vi "Periodic Tasks.vi"(8 "error in":errorcluster) -> ()   [LabVIEW 2020]
doc: "This VI runs in parallel to other robot code. It can contain as many user-defined periodic loops as you need. These can carry out PID or other sorts of timed response."
uses:
  <vilib>/Rock Robotics/WPI/ThirdParty/Phoenix-LabVIEW/Motor Controller/Get/CTRE_Phoenix_MotorController_GetSupplyAndStatorCurrent_Enhanced.vi
  <vilib>/Rock Robotics/WPI/ThirdParty/Phoenix-LabVIEW/Motor Controller/Get/CTRE_Phoenix_MotorController_GetSelectedSensorData.vi
  <vilib>/Rock Robotics/WPI/ThirdParty/Phoenix-LabVIEW/Motor Controller/Get/CTRE_Phoenix_MotorController_GetTemperature.vi
  <vilib>/nisyscfg/nisyscfg.lvlib
  <resource>/objmgr/nisysapi.rc
  <vilib>/NI_Real-Time Target Support.lvlib
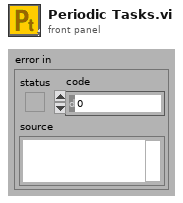
[diagram p1: front panel]
types:
  T1 = typedef "WPI_MotorControlDeviceRef.ctl" = cluster{"DeviceStatus":errorcluster, "Type":T2, "PWM":cluster{"PWM Channel":T3, "DeadBand":T4}, "CAN":cluster{"Device Number":u8, "SetOutput VI Ref":variant, "GetOutput VI Ref":variant, "Enable VI Ref":variant, "Disable VI Ref":variant, "Data":variant}, "Invert":bool, "DIO PWM":cluster{"PWM \"Enable\" Channel":T3, "DIOChannel":T5, "PWM Rate":dbl}}
  T2 = typedef "WPI_MotorControlType.ctl" = enum16{"PWM", "CAN", "DIO PWM"}
  T3 = typedef "FPGA_DIOPWMChannel.ctl" = enum8{"PWM 0", "PWM 1", "PWM 2", "PWM 3", "PWM 4", "PWM 5", "PWM 6", "PWM 7", "PWM 8", "PWM 9", "PWM MXP 0", "PWM MXP 1", "PWM MXP 2", "PWM MXP 3", "PWM MXP 4", "PWM MXP 5", "PWM MXP 6", "PWM MXP 7", "PWM MXP 8", "PWM MXP 9", "Invalid"}
  T4 = typedef "WPI_PWMDeadband.ctl" = cluster{"Name":string, "maxPositivePwm":i32, "minPositivePwm":i32, "centerPwm":i32, "maxNegativePwm":i32, "minNegativePwm":i32, "angularRange":u16}
  T5 = typedef "FPGA_DIOChannel.ctl" = enum8{"DIO 0", "DIO 1", "DIO 2", "DIO 3", "DIO 4", "DIO 5", "DIO 6", "DIO 7", "DIO 8", "DIO 9", "DIO MXP 0", "DIO MXP 1", "DIO MXP 2", "DIO MXP 3", "DIO MXP 4", "DIO MXP 5", "DIO MXP 6", "DIO MXP 7", "DIO MXP 8", "DIO MXP 9", "DIO MXP 10", "DIO MXP 11", "DIO MXP 12", "DIO MXP 13", "DIO MXP 14", "DIO MXP 15", "SPI Port CS1", "SPI Port CS2", "SPI Port CS3", "SPI Port MISO", "SPI Port MOSI", "Invalid"}
  T6 = typedef "NI_Real-Time Target Support.lvlib/RT CPU Load.ctl" = cluster{"Total (%)":dbl, "Time Critical (%)":dbl, "Timed Structures (%)":dbl, "High (%)":dbl, "Above Normal (%)":dbl, "Normal (%)":dbl, "Background (%)":dbl, "Idle (%)":dbl, "ISR (%)":dbl}
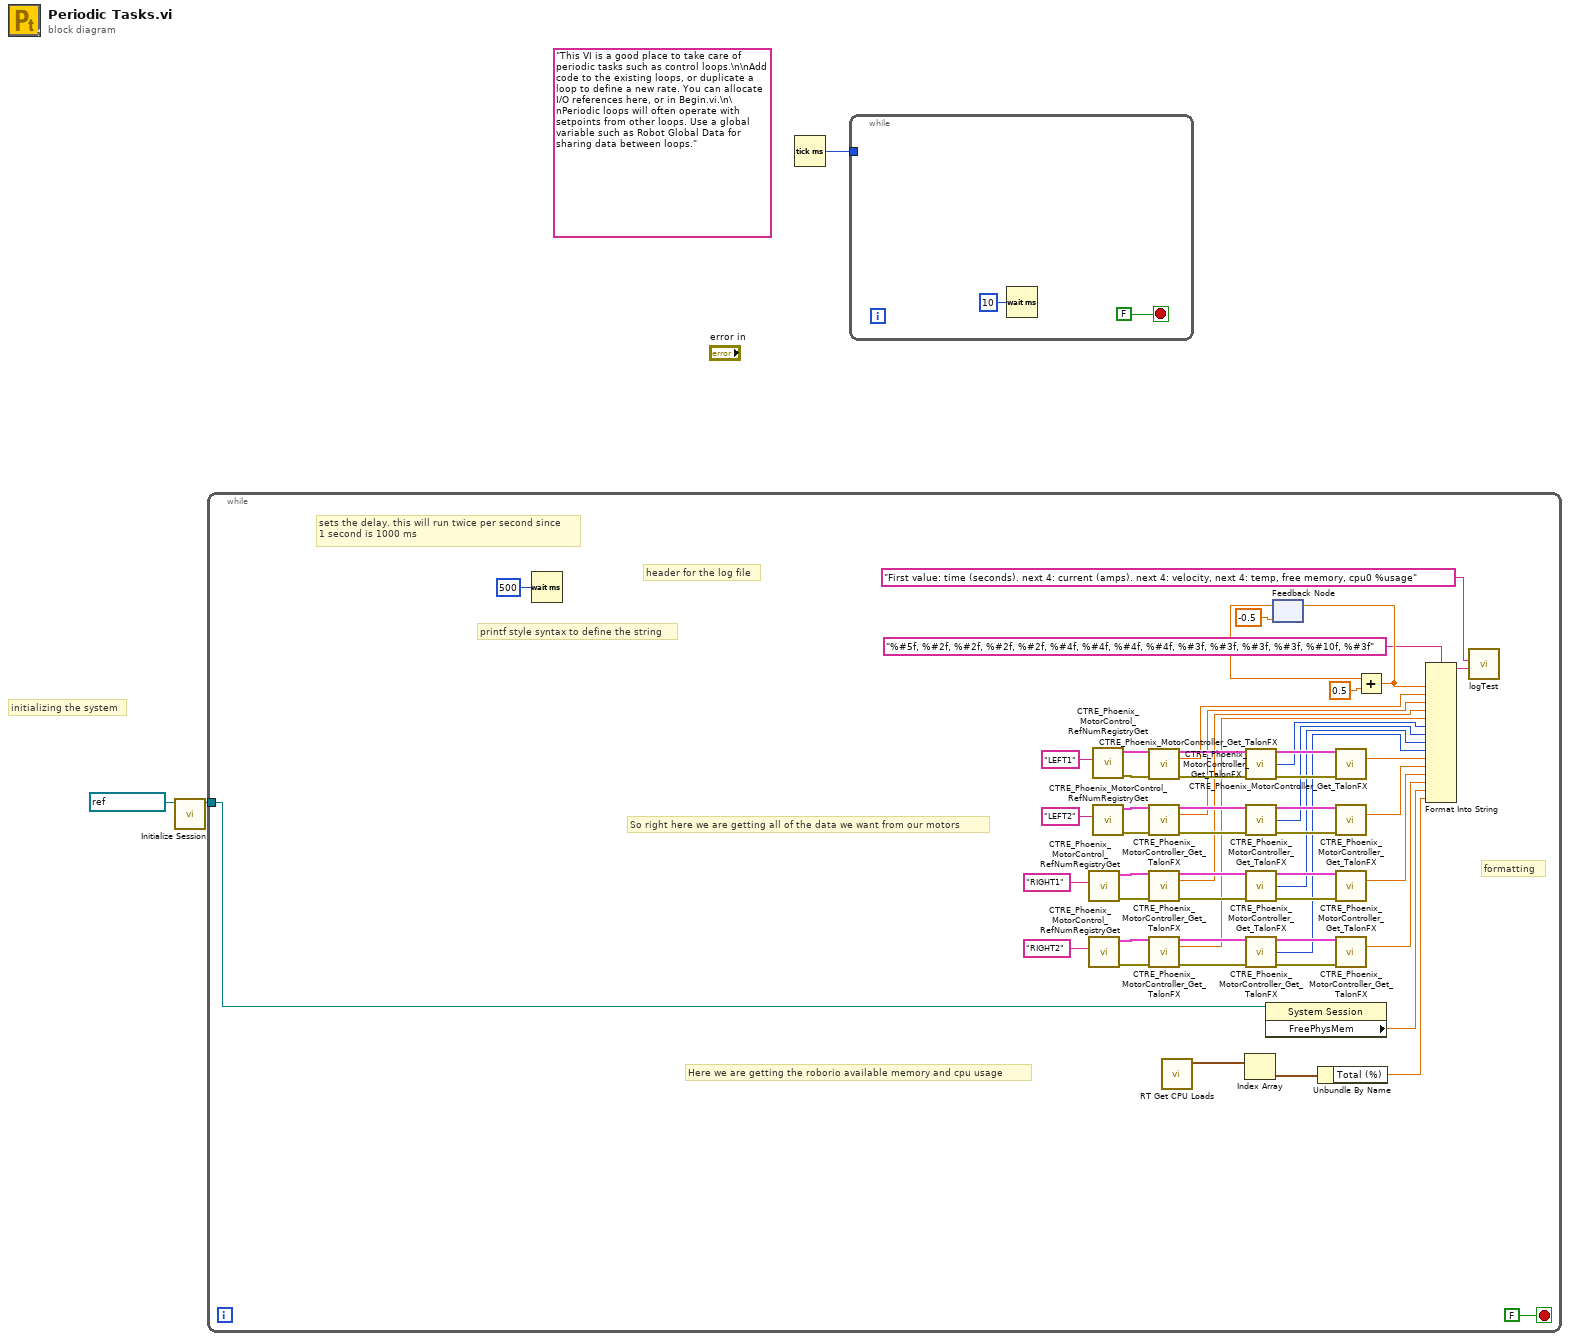
[diagram p0: block diagram]
diagram:
  (unwired) "This VI is a good place to take care of periodic tasks such as control loops.\n\nAdd code to the existing loops, or duplicate a loop to define a new rate. You can allocate I/O references here, or in Begin.vi.\n\nPeriodic loops will often operate with setpoints from other loops. Use a global variable such as Robot Global Data for sharing data between loops."
  # "initializing the system"
  n1 = call <vilib>:"Initialize Session.vi"("Target (localhost)"=refnum<k21> "localhost") -> ("Session out"=w1:refnum<k21>)  [unwired: 9 in, 1 out]
  n2 = while {
    tunnel: w1 -> [w9]
    stop <- FALSE stop-if-true
    # "formatting"
    # "sets the delay. this will run twice per second since\n1 second is 1000 ms"
    # "header for the log file"
    # "printf style syntax to define the string"
    # "Here we are getting the roborio available memory and cpu usage"
    # "So right here we are getting all of the data we want from our motors"
    n3 = Wait (ms)(milliseconds to wait=u32 500) -> ()  [unwired: 1 out]
    n4 = call <vilib>:"CTRE_Phoenix_MotorControl_RefNumRegistryGet.vi"("refnum name"="RIGHT1") -> ("error out"=w40:errorcluster, "PhoenixMotorControlDevRef"=w41:T1)  [unwired: 9 in]
    n5 = call <vilib>:"CTRE_Phoenix_MotorControl_RefNumRegistryGet.vi"("refnum name"="RIGHT2") -> ("error out"=w38:errorcluster, "PhoenixMotorControlDevRef"=w39:T1)  [unwired: 9 in]
    n6 = call <vilib>:"CTRE_Phoenix_MotorControl_RefNumRegistryGet.vi"("refnum name"="LEFT1") -> ("error out"=w44:errorcluster, "PhoenixMotorControlDevRef"=w45:T1)  [unwired: 9 in]
    n7 = call <vilib>:"CTRE_Phoenix_MotorControl_RefNumRegistryGet.vi"("refnum name"="LEFT2") -> ("error out"=w42:errorcluster, "PhoenixMotorControlDevRef"=w43:T1)  [unwired: 9 in]
    n8 = call-poly <vilib>:"CTRE_Phoenix_MotorController_Get_TalonFX.vi"("PhoenixMotorControlDevRef"=w45, "error in"=w44) -> ("PhoenixMotorControlDevRef"=w37:T1, "Supply Current"=w21:dbl, "error out"=w36:errorcluster)  [unwired: 10 in, 1 out]
    n9 = call-poly <vilib>:"CTRE_Phoenix_MotorController_Get_TalonFX.vi"("PhoenixMotorControlDevRef"=w43, "error in"=w42) -> ("PhoenixMotorControlDevRef"=w35:T1, "Supply Current"=w20:dbl, "error out"=w34:errorcluster)  [unwired: 10 in, 1 out]
    n10 = call-poly <vilib>:"CTRE_Phoenix_MotorController_Get_TalonFX.vi"("PhoenixMotorControlDevRef"=w41, "error in"=w40) -> ("PhoenixMotorControlDevRef"=w33:T1, "Supply Current"=w19:dbl, "error out"=w32:errorcluster)  [unwired: 10 in, 1 out]
    n11 = call-poly <vilib>:"CTRE_Phoenix_MotorController_Get_TalonFX.vi"("PhoenixMotorControlDevRef"=w39, "error in"=w38) -> ("PhoenixMotorControlDevRef"=w31:T1, "Supply Current"=w18:dbl, "error out"=w30:errorcluster)  [unwired: 10 in, 1 out]
    n12 = call <vilib>:"RT Get CPU Loads.vi"() -> ("CPU loads"=w6:T6[])  [unwired: 10 in, 1 out]
    n13 = Index Array(array=w6) -> (element=w5:T6)  [unwired: 1 in]
    n14 = call-poly <vilib>:"CTRE_Phoenix_MotorController_Get_TalonFX.vi"("PhoenixMotorControlDevRef"=w37, "error in"=w36) -> ("PhoenixMotorControlDevRef"=w29:T1, "Velocity (Raw Sensor Units per 100 ms)"=w17:i32, "error out"=w28:errorcluster)  [unwired: 10 in, 1 out]
    n15 = call-poly <vilib>:"CTRE_Phoenix_MotorController_Get_TalonFX.vi"("PhoenixMotorControlDevRef"=w35, "error in"=w34) -> ("PhoenixMotorControlDevRef"=w27:T1, "Velocity (Raw Sensor Units per 100 ms)"=w16:i32, "error out"=w26:errorcluster)  [unwired: 10 in, 1 out]
    n16 = call-poly <vilib>:"CTRE_Phoenix_MotorController_Get_TalonFX.vi"("PhoenixMotorControlDevRef"=w33, "error in"=w32) -> ("PhoenixMotorControlDevRef"=w25:T1, "Velocity (Raw Sensor Units per 100 ms)"=w15:i32, "error out"=w24:errorcluster)  [unwired: 10 in, 1 out]
    n17 = call-poly <vilib>:"CTRE_Phoenix_MotorController_Get_TalonFX.vi"("PhoenixMotorControlDevRef"=w31, "error in"=w30) -> ("PhoenixMotorControlDevRef"=w23:T1, "Velocity (Raw Sensor Units per 100 ms)"=w14:i32, "error out"=w22:errorcluster)  [unwired: 10 in, 1 out]
    n18 = property class="System Session"(reference=w9) -> ("FreePhysMem"=w8:dbl)  [unwired: 1 in, 2 out]
    n19 = feedback #1(-0.5) -> (w53:dbl)
    n20 = Unbundle By Name(w5) -> ("Total (%)"=w4:dbl)
    n21 = call-poly <vilib>:"CTRE_Phoenix_MotorController_Get_TalonFX.vi"("PhoenixMotorControlDevRef"=w29, "error in"=w28) -> ("Temperature (C)"=w13:dbl)  [unwired: 11 in, 2 out]
    n22 = call-poly <vilib>:"CTRE_Phoenix_MotorController_Get_TalonFX.vi"("PhoenixMotorControlDevRef"=w27, "error in"=w26) -> ("Temperature (C)"=w12:dbl)  [unwired: 11 in, 2 out]
    n23 = call-poly <vilib>:"CTRE_Phoenix_MotorController_Get_TalonFX.vi"("PhoenixMotorControlDevRef"=w25, "error in"=w24) -> ("Temperature (C)"=w11:dbl)  [unwired: 11 in, 2 out]
    n24 = call-poly <vilib>:"CTRE_Phoenix_MotorController_Get_TalonFX.vi"("PhoenixMotorControlDevRef"=w23, "error in"=w22) -> ("Temperature (C)"=w10:dbl)  [unwired: 11 in, 2 out]
    n25 = Add(x=w53, y=0.5) -> (x+y=w51:dbl)
    n26 = feedback-in #1(w51) -> ()
    n27 = Format Into String(format string="%#5f, %#2f, %#2f, %#2f, %#2f, %#4f, %#4f, %#4f, %#4f, %#3f, %#3f, %#3f, %#3f, %#10f, %#3f", w51, w21, w20, w19, w18, w17, w16, w15, w14, w13, w12, w11, w10, w8, w4) -> (resulting string=w55:string)  [unwired: 2 in, 1 out]
    n28 = call "logTest.vi"("Input"=w55, "Header"="First value: time (seconds). next 4: current (amps). next 4: velocity, next 4: temp, free memory, cpu0 %usage") -> ()  [unwired: 10 in]
  }
  n29 = Tick Count (ms)() -> (millisecond timer value=w3:u32)
  n30 = while {
    tunnel: w3 -> [_]
    stop <- FALSE stop-if-true
    n31 = Wait (ms)(milliseconds to wait=u32 10) -> ()  [unwired: 1 out]
  }
